vi "convert nanoseconds to timespec.vi"(11 "nanoseconds":i64) -> (3 "timespec":cluster{"sec":u64, "nsec":u64})   [LabVIEW 2013, in "Linux RT Utilities.lvlib"]
uses:
  Linux RT Utilities.lvlib
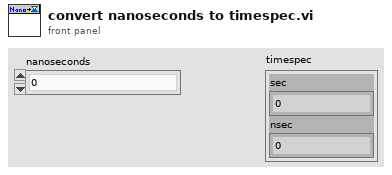
[diagram p1: front panel]
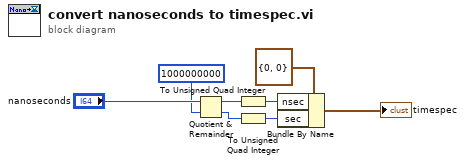
[diagram p0: block diagram]
diagram:
  n1 = Quotient & Remainder(x="nanoseconds", y=i64 1000000000 ("x")) -> (x-y*floor(x/y)=w4:i64, floor(x/y)=w1:i64)
  n2 = To Unsigned Quad Integer(1:w4) -> (0:w3:u64)
  n3 = To Unsigned Quad Integer(1:w1) -> (0:w2:u64)
  n4 = Bundle By Name(cluster=cluster{"sec":u64, "nsec":u64} {"sec"=0, "nsec"=0} ("timespec"), "nsec"=w3, "sec"=w2) -> (→"timespec":cluster{"sec":u64, "nsec":u64})
